vi "GetVerbosity.vi"(8 "error in (no error)":errorcluster) -> (0 "error out":errorcluster, 2 "Found":bool, 3 "Verbosity":T1=enum."INFO")   [LabVIEW 2026, in "Lumberjack.lvlib"]
uses:
  Lumberjack.lvlib
  TypeDefs/Severity.ctl
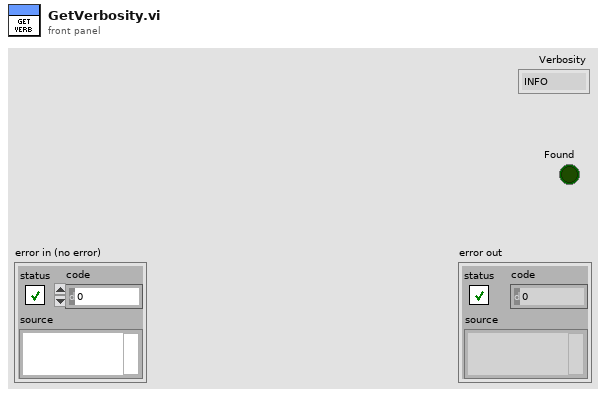
[diagram p1: front panel]
types:
  T1 = typedef "Lumberjack.lvlib/Severity.ctl" = enum16{"OFF", "FATAL", "ERROR", "WARN", "INFO", "DEBUG", "TRACE", "ALL"}
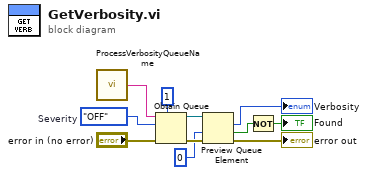
[diagram p0: block diagram]
diagram:
  w6 = Severity."OFF"  # Severity
  n1 = call "ProcessVerbosityQueueName.vi"() -> ("processVerbosityQueueName"=w7:string)
  n2 = Obtain Queue(max queue size (-1, unlimited)=1, name (unnamed)=w7, element data type=w6, error in (no error)="error in (no error)") -> (queue out=w8:refnum<queue>, error out=w10:errorcluster)  [unwired: 1 in, 1 out]
  n3 = Preview Queue Element(queue=w8, timeout in ms (-1)=0, error in (no error)=w10) -> (element=→"Verbosity":T1, timed out?=w3:bool, error out=→"error out":errorcluster)  [unwired: 1 out]
  n4 = Not(x=w3) -> (.not. x?=→"Found":bool)
